vi "FindPosForItem.vi"(0 "reference in":refnum<class "VINode.lvclass">, 1 "SearchItem":string, 2 "AttributesIDs":string[](array[string]), 3 "MethodIDs":string[](array[string]), 5 "error in (no error)":errorcluster) -> (12 "UpperRightPoint":T1 {"y" format="%.2f"; "x" format="%.2f"}, 14 "reference out":refnum<class "VINode.lvclass">, 15 "LeftPoint":T1 {"y" format="%.2f"; "x" format="%.2f"}, 16 "CenterPoint":T1 {"y" format="%.2f"; "x" format="%.2f"}, 17 "RightPoint":T1 {"y" format="%.2f"; "x" format="%.2f"}, 18 "UpperLeftPoint":T1 {"y" format="%.2f"; "x" format="%.2f"}, 19 "error out":errorcluster)   [LabVIEW 2020, in "VINode.lvclass"]
doc: "public void draw(Graphics2D g2, Point2D p, Point2D q)"
uses:
  <resource>/Framework/Providers/Open_GDS/UML/VINode_class/VINode.lvclass
  C:/Program Files (x86)/National Instruments/LabVIEW 2020/resource/Framework/Providers/Open_GDS/UML/RectangularNode_class/RectangularNode.lvclass
  <resource>/Framework/Providers/Open_GDS/UML/General/Point/Point Point2D.ctl
  <resource>/Framework/Providers/Open_GDS/UML/General/Rectangle/Rectangle Rectangle2D.ctl
  <resource>/Framework/Providers/Open_GDS/UML/MultiLineString_class/MultiLineString.lvclass
  <resource>/Framework/Providers/Open_GDS/UML/RectangularNode_class/RectangularNode.lvclass
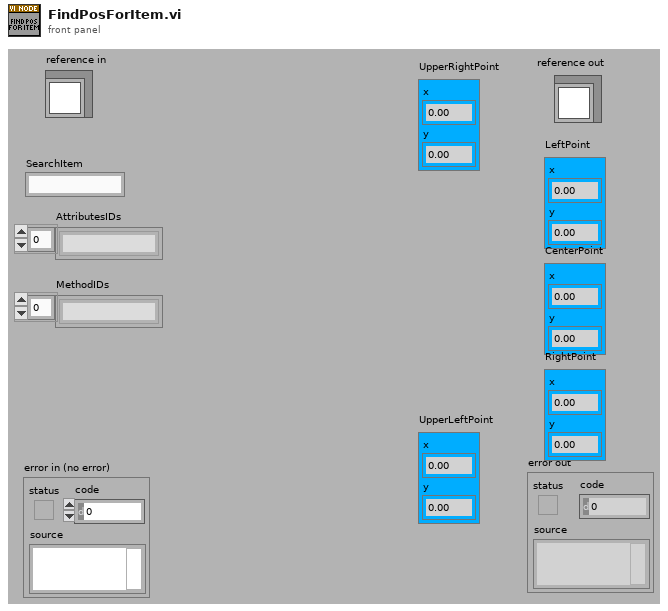
[diagram p1: front panel]
types:
  T1 = typedef "Point Point2D.ctl" = cluster{"x":dbl, "y":dbl}
  T2 = typedef "Rectangle Rectangle2D.ctl" = cluster{"x":dbl, "y":dbl, "width":dbl, "height":dbl}
  T3 = typedef "VINode.lvclass/ObjectAttributes.ctl" = cluster{"midHeight":dbl, "botHeight":dbl, "Name":refnum<class "MultiLineString.lvclass">, "DEFAULT_COMPARTMENT_HEIGHT":i32, "DEFAULT_WIDTH":i32, "DEFAULT_HEIGHT":i32, "VIPath":path, "Description":refnum<class "MultiLineString.lvclass">, "ShowDescription":bool}
  T4 = typedef "RectangularNode.lvclass/ObjectAttributes.ctl" = cluster{"bounds":T2}
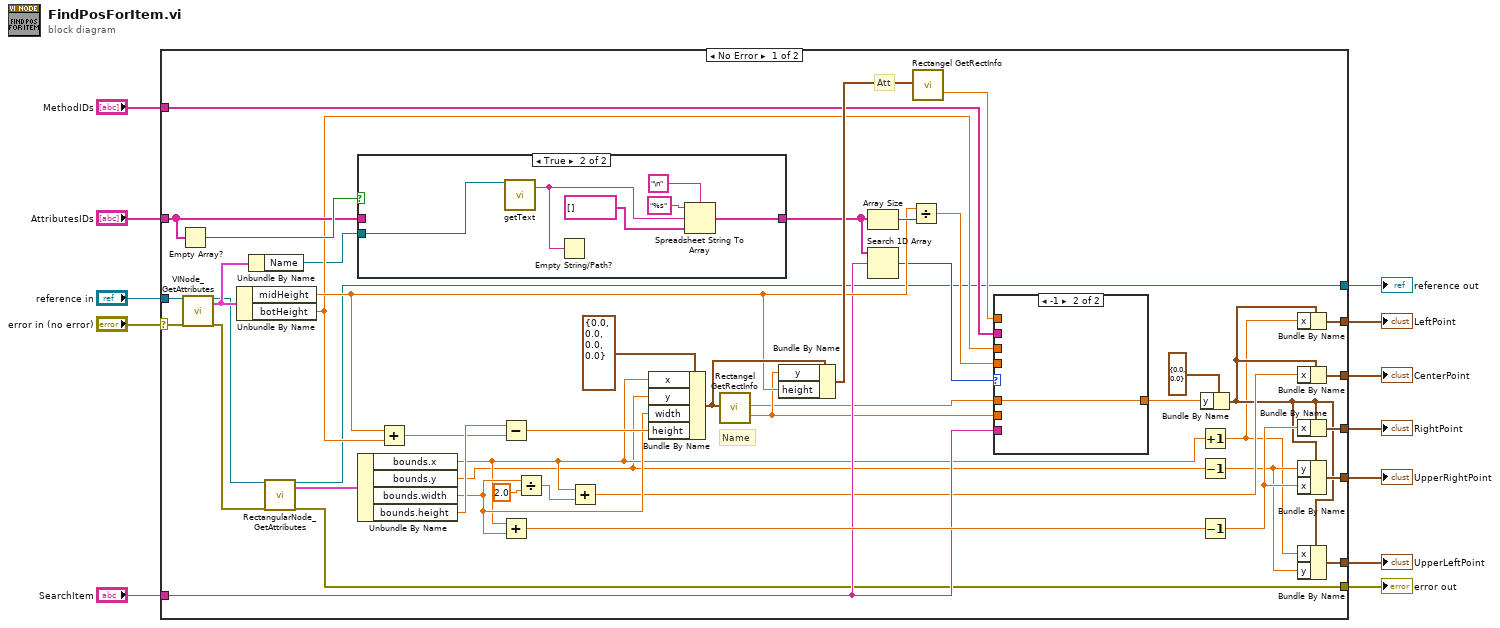
[diagram p0: block diagram]
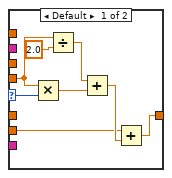
[diagram p3: hidden frame]
diagram:
  n1 = case shown="No Error" "error in (no error)" {
    selector: "error in (no error)" -> [w57 w75]
    tunnel: "reference in" -> [w58 w76]
    tunnel: [w16 w75] -> w11
    tunnel: [w15 w76] -> w10
    tunnel: "SearchItem" -> [w34 _]
    tunnel: "AttributesIDs" -> [w44 _]
    tunnel: [w41 _] -> w6
    tunnel: [w39 _] -> w5
    tunnel: [w38 _] -> w4
    tunnel: "MethodIDs" -> [w35 _]
    tunnel: [w24 _] -> w2
    tunnel: [w22 _] -> w1
    frame No Error {
      # "Att"
      # "Name"
      n2 = Empty Array?(array=w44) -> (empty?=w45:bool)
      n3 = call <resource>:"VINode_GetAttributes.vi"("reference in"=w58, "error in (no error)"=w57) -> ("reference out"=w18:refnum<class "VINode.lvclass">, "Data"=w19:T3, "error out"=w17:errorcluster)  [unwired: 1 in, 14 out]
      n4 = Unbundle By Name(w19) -> ("midHeight"=w48:dbl, "botHeight"=w30:dbl)
      n5 = Unbundle By Name(w19) -> ("Name"=w13:refnum<class "MultiLineString.lvclass">)
      n6 = call <resource>:"RectangularNode_GetAttributes.vi"("reference in"=w18, "error in (no error)"=w17) -> ("reference out"=w15:refnum<class "VINode.lvclass">, "Data"=w14:T4, "error out"=w16:errorcluster)  [unwired: 14 in, 1 out]
      n7 = case shown="True" w45 {
        tunnel: [w59 w61] -> w50
        tunnel: w13 -> [_ w60]
        tunnel: w44 -> [w59 _]
        frame False {
        }
        frame True {
          n8 = call-dynamic "getText.vi"("reference"=w60) -> ("text"=w62:string)  [unwired: 1 in, 17 out]
          n9 = Empty String/Path?(string/path=w62) -> ()  [unwired: 1 out]
          n10 = Spreadsheet String To Array(delimiter (Tab)="\n", format string="%s", spreadsheet string=w62, array type (2D Dbl)=string[] []) -> (array=w61:string[])
        }
      }
      n11 = Unbundle By Name(w14) -> ("bounds.x"=w29:dbl, "bounds.y"=w25:dbl, "bounds.width"=w37:dbl, "bounds.height"=w55:dbl)
      n12 = Add(x=w48, y=w30) -> (x+y=w53:dbl)
      n13 = Subtract(x=w55, y=w53) -> (x-y=w54:dbl)
      n14 = Add(x=w29, y=w37) -> (x+y=w36:dbl)
      n15 = Divide(x=w37, y=2.0) -> (x/y=w28:dbl)
      n16 = Add(x=w29, y=w28) -> (x+y=w27:dbl)
      n17 = Bundle By Name(cluster=T2 {"x"=0.0, "y"=0.0, "width"=0.0, "height"=0.0} ("points"), "x"=w29, "y"=w25, "width"=w37, "height"=w54) -> (w52:T2)
      n18 = call <resource>:"Rectangel GetRectInfo.vi"("bounds"=w52) -> ("centerY"=w32:dbl, "maxY"=w33:dbl)  [unwired: 1 in, 16 out]
      n19 = Bundle By Name(cluster=w52, "y"=w33, "height"=w48) -> (w51:T2)
      n20 = Array Size(array=w50) -> (size(s)=w49:i32)
      n21 = Search 1D Array(1D array=w50, element=w34) -> (index of element=w46:i32)  [unwired: 1 in]
      n22 = Divide(x=w48, y=w49) -> (x/y=w47:dbl)
      n23 = call <resource>:"Rectangel GetRectInfo.vi"("bounds"=w51) -> ("maxY"=w31:dbl)  [unwired: 1 in, 17 out]
      n24 = case shown="-1" w46 {
        selector: w46 -> [w73 _]
        tunnel: w47 -> [w71 _]
        tunnel: [w66 w74] -> w42
        tunnel: w35 -> [_ _]
        tunnel: w34 -> [_ _]
        tunnel: w33 -> [w67 _]
        tunnel: w32 -> [_ w74]
        tunnel: w31 -> [_ _]
        tunnel: w30 -> [_ _]
        frame Default {
          n25 = Multiply(x=w71, y=w73) -> (x*y=w72:dbl)
          n26 = Divide(x=w71, y=2.0) -> (x/y=w69:dbl)
          n27 = Add(x=w69, y=w72) -> (x+y=w68:dbl)
          n28 = Add(x=w67, y=w68) -> (x+y=w66:dbl)
        }
        frame -1 {
        }
      }
      n29 = Increment(x=w29) -> (x+1=w20:dbl)
      n30 = Decrement(x=w25) -> (x-1=w21:dbl)
      n31 = Decrement(x=w36) -> (x-1=w26:dbl)
      n32 = Bundle By Name(cluster=T1 {"x"=0.0, "y"=0.0} ("LeftPoint"), "y"=w42) -> (w23:T1)
      n33 = Bundle By Name(cluster=w23, "x"=w20) -> (w41:T1)
      n34 = Bundle By Name(cluster=w23, "x"=w27) -> (w39:T1)
      n35 = Bundle By Name(cluster=w23, "x"=w26) -> (w38:T1)
      n36 = Bundle By Name(cluster=w23, "y"=w21, "x"=w26) -> (w24:T1)
      n37 = Bundle By Name(cluster=w23, "x"=w20, "y"=w21) -> (w22:T1)
    }
    frame Error {
    }
  }
  "reference out" <- w10
  "error out" <- w11
  "LeftPoint" <- w6
  "CenterPoint" <- w5
  "RightPoint" <- w4
  "UpperRightPoint" <- w2
  "UpperLeftPoint" <- w1
